vi "TraverseGetSetups.vi"(2 "Speed Factor":dbl=1.0 min=0.1 max=5.0 format="%.2f", 3 "Traverse Name":string="EnFlo Tunnel", 4 "Home":T1) -> (0 "Matched Configurations":T2[](array[typedef]) {"Static Drive Configuration"."Indexer Mode  (FSA)" items=["Incremental", "Absolute"]; "Static Drive Configuration"."Buffer at Stop (SSH)" items=["Clear buffer", "Save and Continue"]; "Static Drive Configuration"."Buffer at Limit (SSG)" items=["Clear buffer", "Save and Continue"]; "Static Drive Configuration"."RS232 Echo Control (SSA)" items=["Echo ON", "Echo OFF"]; "Static Drive Configuration"."Reference edge of Home (OSH)" items=["CW", "CCW"]; "Static Drive Configuration"."Encoder Z for Home (OSD)" items=["Don't use", "Enable"]; "Static Drive Configuration"."Home Switch Sense (OSC)" items=["Normally Open", "Normally Closed"]; "Static Drive Configuration"."Home Position (OSB)" items=["Anywhere in Switch", "Edge of Switch"]; "Static Drive Configuration"."Limit Switch Sense (OSA)" items=["Normally Closed", "Normally Open"]; "Static Drive Configuration"."Limit Disable (LD)" items=["Both Enabled", "CW Disabled", "CCW Disabled", "Both Disabled"]; "Static Drive Configuration"."Stall Detect (FSH)" items=["Disable", "Enable"]; "Static Drive Configuration"."OP2 in Deadband (FSG)" items=["Don't Use", "ACTIVATE"]; "Static Drive Configuration"."Stop on Trigger 3 (FSF)" items=["Ignore", "STOP!"]; "Static Drive Configuration"."Activate OP1 on stall (FSE)" items=["Do not Activate", "ACTIVATE!"]; "Static Drive Configuration"."Stop on Stall (FSD)" items=["Continue", "STOP"]; "Static Drive Configuration"."Position Maintenance (FSC)" items=["Disabled", "Enabled"]; "Static Drive Configuration"."Step Mode  (FSB)" items=["Motor", "Encoder"]; "Static Drive Configuration"."Encoder Resolution (ER)" min=1 max=50000; "Static Drive Configuration"."Dead Band Window (DW)" min=0 max=999999999; "Static Drive Configuration"."Dead Band (DB)" min=0 max=999999999; "Static Drive Configuration"."Correction Gain % (CG)" items=["n/a", "12.5", "25", "37.5", "50", "62.5", "75", "87.5", "100"]; "Channel Properties"."Current Pos" format="%.2f"; "Channel Properties"."Backlash/Eng units" format="%.2f"; "Channel Properties"."Pulses/rev" format="%.2f"; "Channel Properties"."Pos Tolerance" format="%.2f"; "Channel Properties"."Pulses/unit" format="%.2f"; "Channel Properties"."Acc. Min" format="%.2f"; "Channel Properties"."Acc. Max" format="%.2f"; "Channel Properties"."Vel. Min" format="%.2f"; "Channel Properties"."Vel. Max" format="%.2f"; "Channel Properties"."Acc. Default" format="%.2f"; "Channel Properties"."Vel. Default" format="%.2f"})   [LabVIEW 2014]
uses:
  ~subVIs/AxisConfigCluster.ctl
  ~subVIs/DriveProperties.ctl
  ~subVIs/DriveStaticConfig.ctl
  Anemometry/Anemometry Sub Vis/Controls/Home.ctl
  Anemometry/Anemometry Sub Vis/Globals/Constants_global.vi
  ~subVIs/DriveConfigGlobal.vi
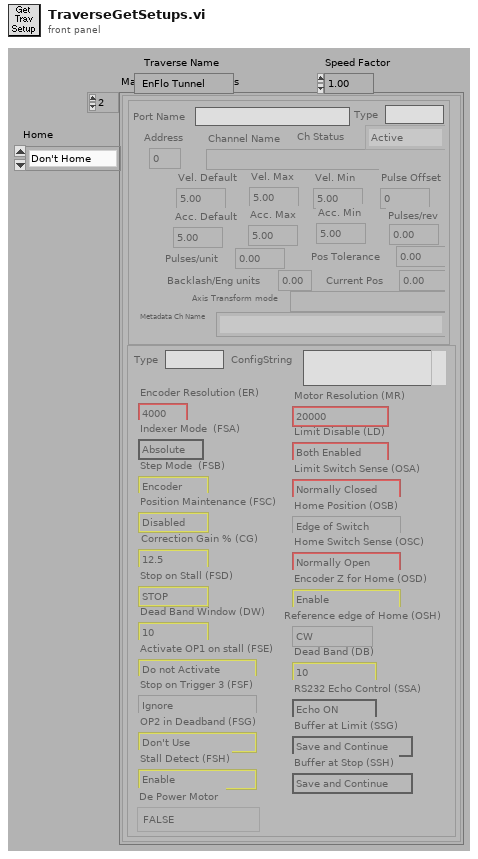
[diagram p1: front panel]
types:
  T1 = typedef "Home.ctl" = enum16{"Don't Home", "Home  +X", "Home  -X", "Home  +Y", "Home  -Y", "Home  +Z", "Home  -Z"}
  T2 = typedef "AxisConfigCluster.ctl" = cluster{"Channel Properties":T3, "Static Drive Configuration":T4}
  T3 = typedef "DriveProperties.ctl" = cluster{"Channel Name":string, "Vel. Default":dbl, "Acc. Default":dbl, "Vel. Max":dbl, "Vel. Min":dbl, "Acc. Max":dbl, "Acc. Min":dbl, "Pulses/unit":dbl, "Address":u8, "Pulse Offset":i32, "Pos Tolerance":dbl, "Pulses/rev":dbl, "Backlash/Eng units":dbl, "Current Pos":dbl, "Ch Status":enum16{"Active", "Offline", "Simulate"}, "Port Name":string, "Axis Transform mode":string, "Metadata Ch Name":string, "Type":string}
  T4 = typedef "DriveStaticConfig.ctl" = cluster{"Correction Gain % (CG)":u16, "Dead Band (DB)":i32, "Dead Band Window (DW)":i32, "Encoder Resolution (ER)":i32, "Step Mode  (FSB)":u16, "Position Maintenance (FSC)":u16, "Stop on Stall (FSD)":u16, "Activate OP1 on stall (FSE)":u16, "Stop on Trigger 3 (FSF)":u16, "OP2 in Deadband (FSG)":u16, "Stall Detect (FSH)":u16, "Limit Disable (LD)":u16, "Motor Resolution (MR)":enum16{"200", "400", "1000", "2000", "4000", "5000", "10000", "12800", "18000", "20000", "21600", "25000", "25400", "25600", "36000", "50000", "278528", "425984", "507904", "614400", "655360", "819200", "1024000"}, "Limit Switch Sense (OSA)":u16, "Home Position (OSB)":u16, "Home Switch Sense (OSC)":u16, "Encoder Z for Home (OSD)":u16, "Reference edge of Home (OSH)":u16, "RS232 Echo Control (SSA)":u16, "Buffer at Limit (SSG)":u16, "Buffer at Stop (SSH)":u16, "Indexer Mode  (FSA)":u16, "Type":string, "ConfigString":string, "De Power Motor":enum16{"TRUE", "FALSE"}}
  T5 = enum16{"Load setup from excel file", "Save setup to excel file"}
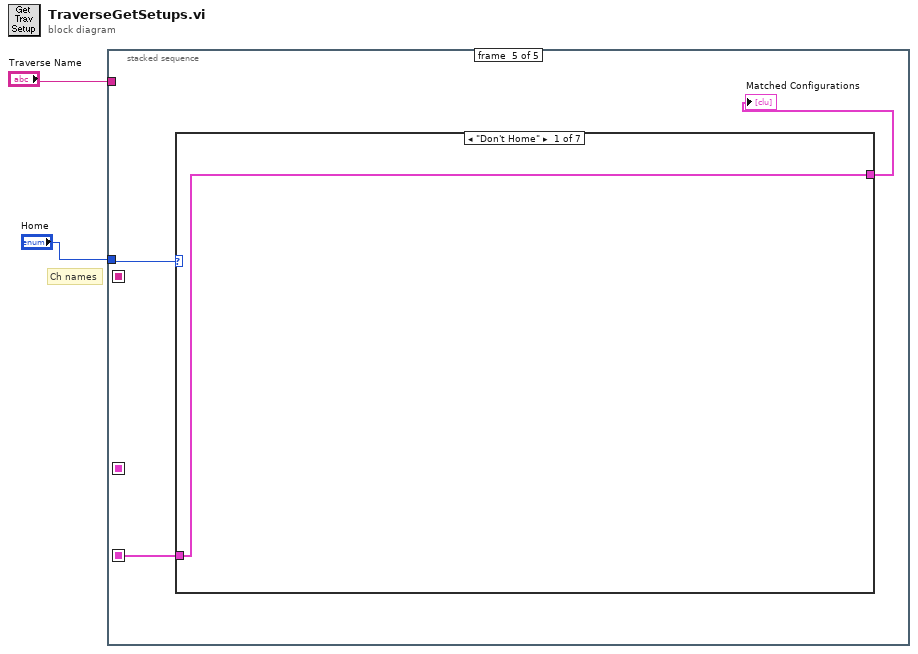
[diagram p0: block diagram]
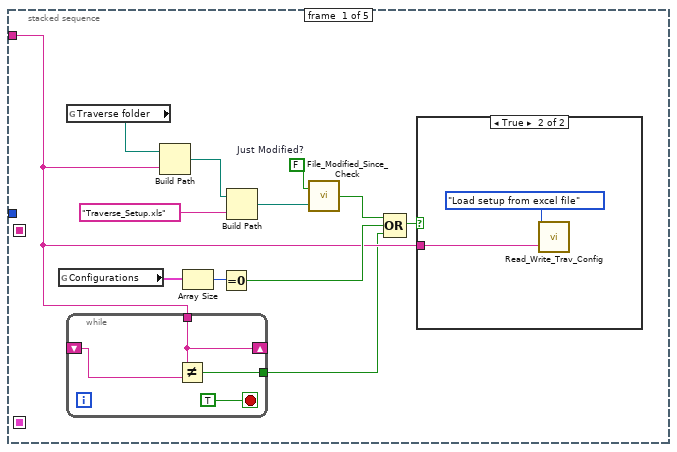
[diagram p2: hidden frame]
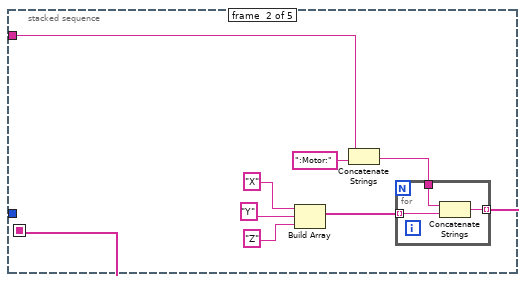
[diagram p4: hidden frame]
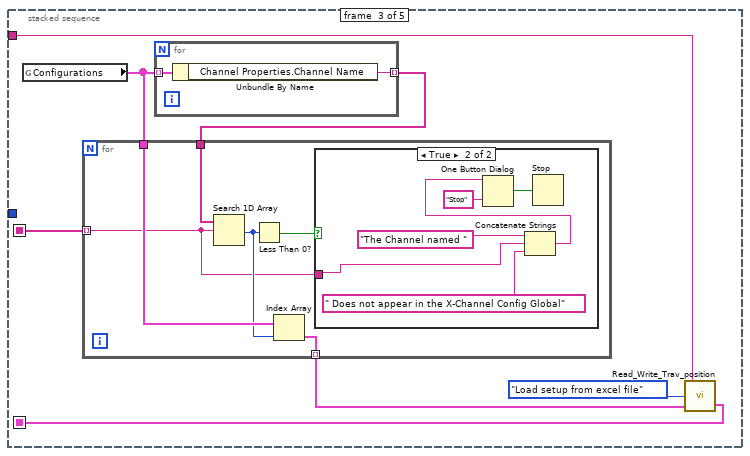
[diagram p5: hidden frame]
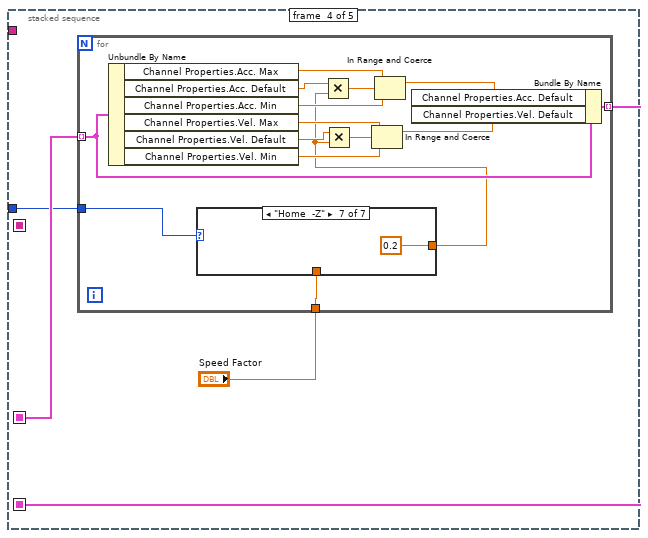
[diagram p7: hidden frame]
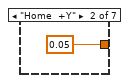
[diagram p9: hidden frame]
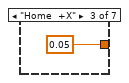
[diagram p10: hidden frame]
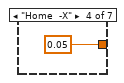
[diagram p11: hidden frame]
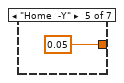
[diagram p12: hidden frame]
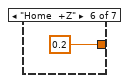
[diagram p13: hidden frame]
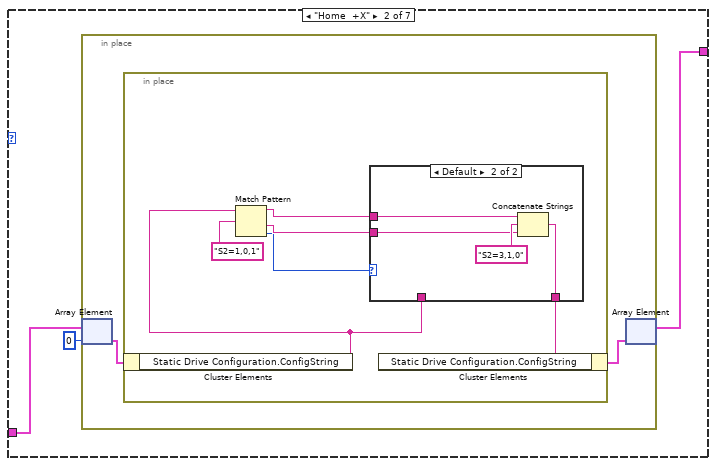
[diagram p14: hidden frame]
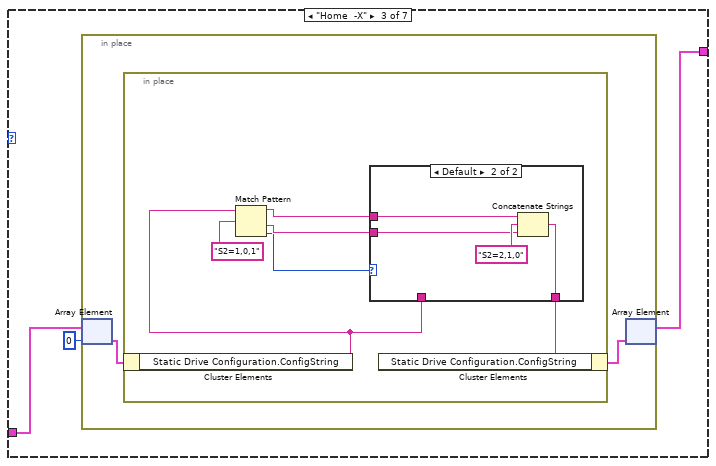
[diagram p16: hidden frame]
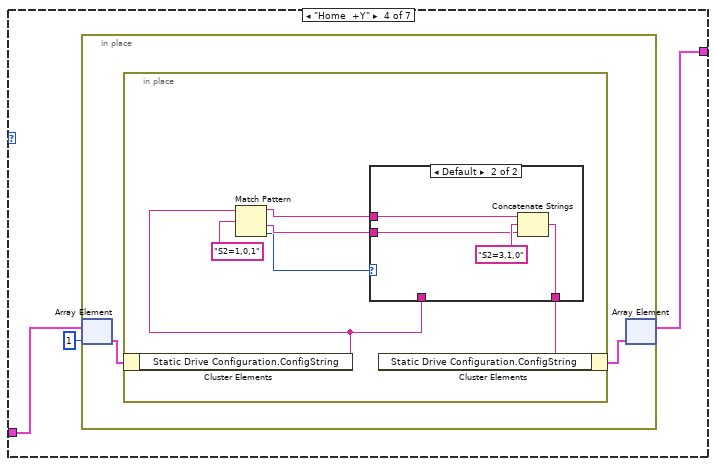
[diagram p18: hidden frame]
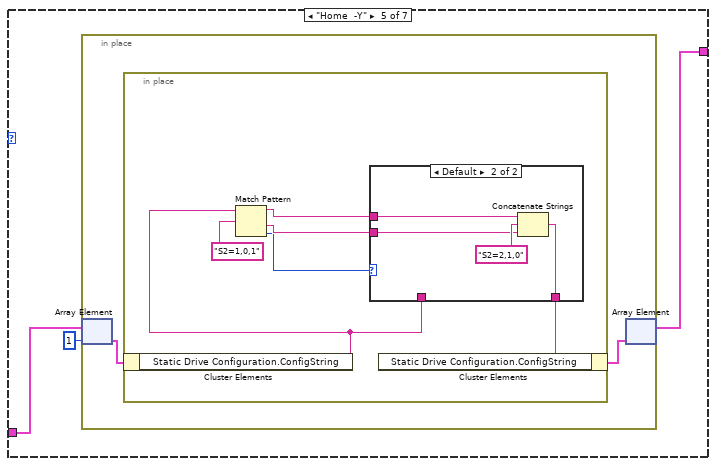
[diagram p20: hidden frame]
diagram:
  # "Ch names"
  n1 = stacked-sequence {
    seq-local: [_ w26 _ _ _] -> [_ _ w37 _ _]
    seq-local: [_ _ w34 _ _] -> [_ _ _ w56 _]
    seq-local: [_ _ _ w53 _] -> [_ _ _ _ w80]
    tunnel: "Traverse Name" -> [w4 w24 w33 _ _]
    tunnel: "Home" -> [_ _ _ w54 w81]
    frame #0 {
      w13 = FALSE  # Just Modified?
      n2 = global read "DriveConfigGlobal.vi" "Configurations"() -> (w12:T2[])
      n3 = global read "Constants_global.vi" "Traverse folder"() -> (w6:path)
      n4 = while {
        shift-right: [w16] -> _
        shift-left: _ -> [w17]
        tunnel: w4 -> [w16]
        tunnel: [w15] -> w3
        stop <- TRUE stop-if-true
        n5 = Not Equal?(x=w16, y=w17) -> (x != y?=w15:bool)
      }
      n6 = Build Path(base path=w6, name or relative path=w4) -> (appended path=w5:path)
      n7 = Array Size(array=w12) -> (size(s)=w11:i32)
      n8 = Equal To 0?(x=w11) -> (x = 0?=w9:bool)
      n9 = Build Path(base path=w5, name or relative path="Traverse_Setup.xls" ("Substring")) -> (appended path=w14:path)
      n10 = call "File_Modified_Since_Check.vi"("Pathname"=w14, "Just Modified?"=w13) -> ("Modified?"=w10:bool)
      n11 = Compound Arithmetic op=OR(w10, w9, w3) -> (w8:bool)
      n12 = case shown="True" w8 {
        tunnel: w4 -> [_ w19]
        frame False {
        }
        frame True {
          n13 = call "Read_Write_Trav_Config.vi"("Traverse Name"=w19, "Mode"=T5."Load setup from excel file") -> ()  [unwired: 1 out]
        }
      }
    }
    frame #1 {
      n14 = Build Array("X", "Y", "Z") -> (w27:string[])
      n15 = Concatenate Strings(w24, ":Motor:") -> (w25:string)
      n16 = for {
        tunnel: w27 -> [w31] mode=indexing
        tunnel: [w29] -> w26 mode=indexing
        tunnel: w25 -> [w30]
        n17 = Concatenate Strings(w30, w31) -> (w29:string)
      }
    }
    frame #2 {
      n18 = global read "DriveConfigGlobal.vi" "Configurations"() -> (w32:T2[])
      n19 = for {
        tunnel: w32 -> [w52] mode=indexing
        tunnel: [w51] -> w38 mode=indexing
        n20 = Unbundle By Name(w52) -> ("Channel Properties.Channel Name"=w51:string)
      }
      n21 = for {
        tunnel: w38 -> [w44]
        tunnel: w32 -> [w42]
        tunnel: [w40] -> w36 mode=indexing
        tunnel: w37 -> [w39] mode=indexing
        n22 = Search 1D Array(1D array=w44, element=w39) -> (index of element=w41:i32)  [unwired: 1 out]
        n23 = Less Than 0?(x=w41) -> (x < 0?=w43:bool)
        n24 = Index Array(array=w42, index=w41) -> (element=w40:T2)
        n25 = case shown="True" w43 {
          tunnel: w39 -> [_ w49]
          frame False {
          }
          frame True {
            n26 = Concatenate Strings("The Channel named " ("message"), w49, " Does not appear in the X-Channel Config Global" ("Input 3")) -> (w45:string)
            n27 = One Button Dialog(message=w45, button name ("OK")="Stop") -> (true=w46:bool)
            n28 = Stop(stop? (T)=w46) -> ()
          }
        }
      }
      n29 = call "Read_Write_Trav_position.vi"("Matched Configurations In"=w36, "Mode"=T5."Load setup from excel file", "Traverse Name"=w33) -> ("Matched Configurations Out"=w34:T2[])  [unwired: 1 out]
    }
    frame #3 {
      n30 = for {
        tunnel: w56 -> [w69] mode=indexing
        tunnel: "Speed Factor" -> [w59]
        tunnel: [w67] -> w53 mode=indexing
        tunnel: w54 -> [w57]
        n31 = Unbundle By Name(w69) -> ("Channel Properties.Acc. Max"=w65:dbl, "Channel Properties.Acc. Default"=w61:dbl, "Channel Properties.Acc. Min"=w64:dbl, "Channel Properties.Vel. Max"=w68:dbl, "Channel Properties.Vel. Default"=w60:dbl, "Channel Properties.Vel. Min"=w71:dbl)
        n32 = case shown="\"Home  -Z\"" w57 {
          tunnel: [w72 0.05 ("Speed Factor") 0.05 ("Speed Factor") 0.05 ("Speed Factor") 0.05 ("Speed Factor") 0.2 ("Speed Factor") 0.2 ("Speed Factor")] -> w58
          tunnel: w59 -> [w72 _ _ _ _ _ _]
          frame "Don't Home" {
          }
          frame "Home  +Y" {
          }
          frame "Home  +X" {
          }
          frame "Home  -X" {
          }
          frame "Home  -Y" {
          }
          frame "Home  +Z" {
          }
          frame "Home  -Z" {
          }
        }
        n33 = Multiply(x=w61, y=w58) -> (x*y=w63:dbl)
        n34 = Multiply(x=w60, y=w58) -> (x*y=w70:dbl)
        n35 = In Range and Coerce(upper limit=w68, x=w70, lower limit=w71) -> (coerced(x)=w66:dbl)  [unwired: 1 out]
        n36 = In Range and Coerce(upper limit=w65, x=w63, lower limit=w64) -> (coerced(x)=w62:dbl)  [unwired: 1 out]
        n37 = Bundle By Name(cluster=w69, "Channel Properties.Acc. Default"=w62, "Channel Properties.Vel. Default"=w66) -> (w67:T2)
      }
    }
    frame #4 {
      n38 = case shown="\"Don't Home\"" w81 {
        tunnel: w80 -> [w82 w85 w101 w117 w133 w149 w165]
        tunnel: [w82 w83 w99 w115 w131 w147 w163] -> w79
        frame "Don't Home" {
        }
        frame "Home  +X" {
          n39 = in-place {
            n40 = in-place-array #1(w85, 0) -> (w87:T2)
            n41 = in-place {
              n42 = in-place-cluster #2(w87) -> ("Static Drive Configuration.ConfigString"=w88:string)
              n43 = Match Pattern(string=w88, regular expression="S2=1,0,1") -> (before substring=w92:string, after substring=w91:string, offset past match=w89:i32)  [unwired: 1 in, 1 out]
              n44 = case shown="Default" w89 {
                tunnel: w92 -> [_ w98]
                tunnel: w91 -> [_ w96]
                tunnel: [w94 w95] -> w90
                tunnel: w88 -> [w94 _]
                frame -1 {
                }
                frame Default {
                  n45 = Concatenate Strings(w98, "S2=3,1,0" ("regular expression"), w96) -> (w95:string)
                }
              }
              n46 = in-place-cluster #2("Static Drive Configuration.ConfigString"=w90) -> (w86:T2)
            }
            n47 = in-place-array #1(w86) -> (w83:T2[])  [unwired: 1 out]
          }
        }
        frame "Home  -X" {
          n48 = in-place {
            n49 = in-place-array #3(w101, 0) -> (w103:T2)
            n50 = in-place {
              n51 = in-place-cluster #4(w103) -> ("Static Drive Configuration.ConfigString"=w104:string)
              n52 = Match Pattern(string=w104, regular expression="S2=1,0,1") -> (before substring=w108:string, after substring=w107:string, offset past match=w105:i32)  [unwired: 1 in, 1 out]
              n53 = case shown="Default" w105 {
                tunnel: w108 -> [_ w114]
                tunnel: w107 -> [_ w112]
                tunnel: [w110 w111] -> w106
                tunnel: w104 -> [w110 _]
                frame -1 {
                }
                frame Default {
                  n54 = Concatenate Strings(w114, "S2=2,1,0" ("regular expression"), w112) -> (w111:string)
                }
              }
              n55 = in-place-cluster #4("Static Drive Configuration.ConfigString"=w106) -> (w102:T2)
            }
            n56 = in-place-array #3(w102) -> (w99:T2[])  [unwired: 1 out]
          }
        }
        frame "Home  +Y" {
          n57 = in-place {
            n58 = in-place-array #5(w117, 1) -> (w119:T2)
            n59 = in-place {
              n60 = in-place-cluster #6(w119) -> ("Static Drive Configuration.ConfigString"=w120:string)
              n61 = Match Pattern(string=w120, regular expression="S2=1,0,1") -> (before substring=w124:string, after substring=w123:string, offset past match=w121:i32)  [unwired: 1 in, 1 out]
              n62 = case shown="Default" w121 {
                tunnel: w124 -> [_ w130]
                tunnel: w123 -> [_ w128]
                tunnel: [w126 w127] -> w122
                tunnel: w120 -> [w126 _]
                frame -1 {
                }
                frame Default {
                  n63 = Concatenate Strings(w130, "S2=3,1,0" ("regular expression"), w128) -> (w127:string)
                }
              }
              n64 = in-place-cluster #6("Static Drive Configuration.ConfigString"=w122) -> (w118:T2)
            }
            n65 = in-place-array #5(w118) -> (w115:T2[])  [unwired: 1 out]
          }
        }
        frame "Home  -Y" {
          n66 = in-place {
            n67 = in-place-array #7(w133, 1) -> (w135:T2)
            n68 = in-place {
              n69 = in-place-cluster #8(w135) -> ("Static Drive Configuration.ConfigString"=w136:string)
              n70 = Match Pattern(string=w136, regular expression="S2=1,0,1") -> (before substring=w140:string, after substring=w139:string, offset past match=w137:i32)  [unwired: 1 in, 1 out]
              n71 = case shown="Default" w137 {
                tunnel: w140 -> [_ w146]
                tunnel: w139 -> [_ w144]
                tunnel: [w142 w143] -> w138
                tunnel: w136 -> [w142 _]
                frame -1 {
                }
                frame Default {
                  n72 = Concatenate Strings(w146, "S2=2,1,0" ("regular expression"), w144) -> (w143:string)
                }
              }
              n73 = in-place-cluster #8("Static Drive Configuration.ConfigString"=w138) -> (w134:T2)
            }
            n74 = in-place-array #7(w134) -> (w131:T2[])  [unwired: 1 out]
          }
        }
        frame "Home  +Z" {
          n75 = in-place {
            n76 = in-place-array #9(w149, 2) -> (w151:T2)
            n77 = in-place {
              n78 = in-place-cluster #10(w151) -> ("Static Drive Configuration.ConfigString"=w152:string)
              n79 = Match Pattern(string=w152, regular expression="S2=1,0,1") -> (before substring=w156:string, after substring=w155:string, offset past match=w153:i32)  [unwired: 1 in, 1 out]
              n80 = case shown="Default" w153 {
                tunnel: w156 -> [_ w162]
                tunnel: w155 -> [_ w160]
                tunnel: [w158 w159] -> w154
                tunnel: w152 -> [w158 _]
                frame -1 {
                }
                frame Default {
                  n81 = Concatenate Strings(w162, "S2=3,1,0" ("regular expression"), w160) -> (w159:string)
                }
              }
              n82 = in-place-cluster #10("Static Drive Configuration.ConfigString"=w154) -> (w150:T2)
            }
            n83 = in-place-array #9(w150) -> (w147:T2[])  [unwired: 1 out]
          }
        }
        frame "Home  -Z" {
          n84 = in-place {
            n85 = in-place-array #11(w165, 2) -> (w167:T2)
            n86 = in-place {
              n87 = in-place-cluster #12(w167) -> ("Static Drive Configuration.ConfigString"=w168:string)
              n88 = Match Pattern(string=w168, regular expression="S2=1,0,1") -> (before substring=w172:string, after substring=w171:string, offset past match=w169:i32)  [unwired: 1 in, 1 out]
              n89 = case shown="Default" w169 {
                tunnel: w172 -> [_ w178]
                tunnel: w171 -> [_ w176]
                tunnel: [w174 w175] -> w170
                tunnel: w168 -> [w174 _]
                frame -1 {
                }
                frame Default {
                  n90 = Concatenate Strings(w178, "S2=3,1,0" ("regular expression"), w176) -> (w175:string)
                }
              }
              n91 = in-place-cluster #12("Static Drive Configuration.ConfigString"=w170) -> (w166:T2)
            }
            n92 = in-place-array #11(w166) -> (w163:T2[])  [unwired: 1 out]
          }
        }
      }
      "Matched Configurations" <- w79
    }
  }
